vi "Get Timestamp Components.vi"() -> ()   [LabVIEW 2014]
uses:
  <vilib>/Utility/miscctls.llb/LVDateTimeRec.ctl
panel:
  out "output cluster":T1
  out "date time rec":T1
  out "current time":timestamp
  out "resulting string":string
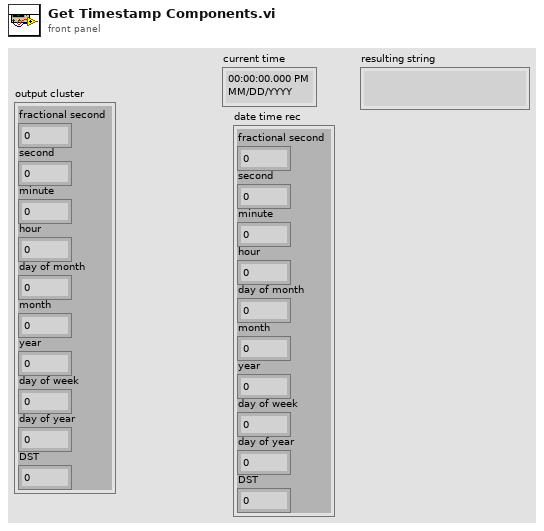
[diagram p1: front panel]
types:
  T1 = typedef "LVDateTimeRec.ctl" = cluster{"fractional second":dbl, "second":i32, "minute":i32, "hour":i32, "day of month":i32, "month":i32, "year":i32, "day of week":i32, "day of year":i32, "DST":i32}
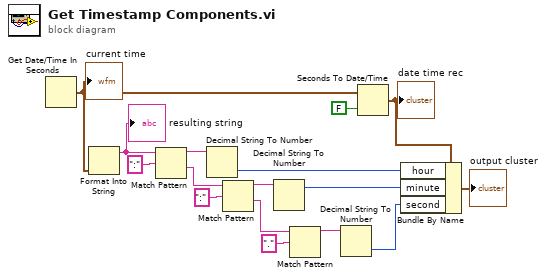
[diagram p0: block diagram]
diagram:
  n1 = Get Date/Time In Seconds() -> (seconds since 1Jan1904=w16:timestamp)
  "current time" <- w16
  n2 = Format Into String(w16) -> (resulting string=w14:string)  [unwired: 3 in, 1 out]
  "resulting string" <- w14
  n3 = Match Pattern(string=w14, regular expression=":") -> (before substring=w11:string, after substring=w8:string)  [unwired: 1 in, 2 out]
  n4 = Decimal String To Number(string=w11) -> (number=w10:i32)  [unwired: 2 in, 1 out]
  n5 = Match Pattern(string=w8, regular expression=":") -> (before substring=w7:string, after substring=w4:string)  [unwired: 1 in, 2 out]
  n6 = Decimal String To Number(string=w7) -> (offset past number=w6:i32)  [unwired: 2 in, 1 out]
  n7 = Match Pattern(string=w4, regular expression=".") -> (before substring=w2:string)  [unwired: 1 in, 3 out]
  n8 = Decimal String To Number(string=w2) -> (number=w1:i32)  [unwired: 2 in, 1 out]
  n9 = Seconds To Date/Time(time stamp (now)=w16, to UTC (F)=FALSE) -> (date time rec=w12:T1)
  "date time rec" <- w12
  n10 = Bundle By Name(cluster=w12, "hour"=w10, "minute"=w6, "second"=w1) -> (→"output cluster":T1)
